vi "DataColumnHead.vi"(8 "error in (no error)":errorcluster caption="错误输入（无错误）", 11 "XYPlot 输入":refnum<class "XYPlot.lvclass">) -> (0 "error out":errorcluster caption="错误输出", 2 "首行":string[](array[string]), 3 "XYPlot 输出":refnum<class "XYPlot.lvclass">)   [LabVIEW 2018, in "DataDisplay.lvlib" / "XYPlot.lvclass"]
uses:
  XYPlot.lvclass
  XYPlot.lvclass/XYPlot.ctl
  SubVI/DD_Parameter.vi
  DataDisplay.lvlib
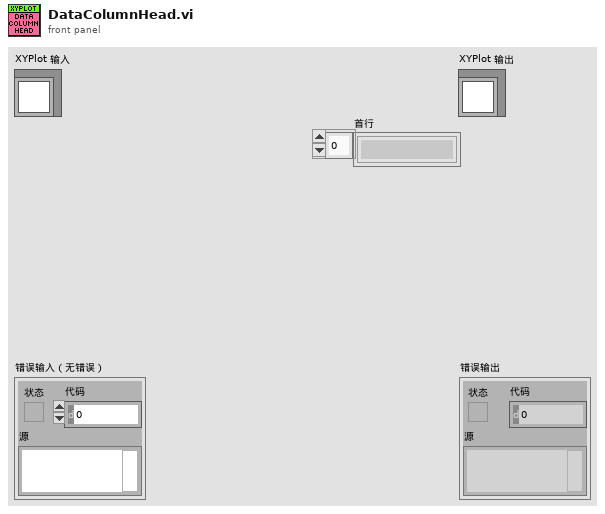
[diagram p1: front panel]
types:
  T1 = typedef "DataDisplay.lvlib/DD_ChannelInfo.ctl" = cluster{"名称":string, "单位":string, "数据类型":enum16{"Real", "Int"}, "趋势线":enum16{"N/A", "X", "Y"}}
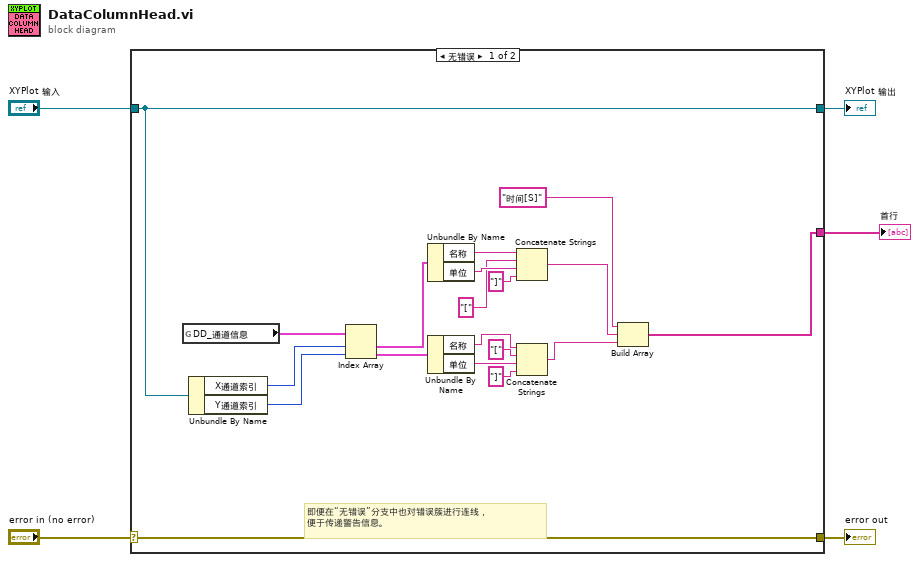
[diagram p0: block diagram]
diagram:
  n1 = case shown="无错误" "error in (no error)" {
    selector: "error in (no error)" -> [w24 w26]
    tunnel: [w24 w26] -> w4
    tunnel: [w23 w25] -> w2
    tunnel: "XYPlot 输入" -> [w23 w25]
    tunnel: [w8 _] -> w1
    frame No Error {
      # "即便在“无错误”分支中也对错误簇进行连线，\n便于传递警告信息。"
      n2 = global read "DD_Parameter.vi" "DD_通道信息"() -> (w22:T1[])
      n3 = Unbundle By Name(w23) -> ("X通道索引"=w21:i32, "Y通道索引"=w20:i32)
      n4 = Index Array(array=w22, index #1=w21, index #2=w20) -> (element #1=w19:T1, element #2=w14:T1)
      n5 = Unbundle By Name(w19) -> ("名称"=w18:string, "单位"=w17:string)
      n6 = Unbundle By Name(w14) -> ("名称"=w7:string, "单位"=w11:string)
      n7 = Concatenate Strings(w18, "[" ("字符串"), w17, "]" ("字符串")) -> (w9:string)
      n8 = Concatenate Strings(w7, "[" ("字符串"), w11, "]" ("字符串")) -> (w6:string)
      n9 = Build Array("时间[S]", w9, w6) -> (w8:string[])
    }
    frame Error {
    }
  }
  "error out" <- w4
  "XYPlot 输出" <- w2
  "首行" <- w1
